vi "Create Evaluation String.vi"(8 "error in (no error)":errorcluster, 10 "Evaluation String":string, 11 "String in":refnum<class "String.lvclass">) -> (0 "error out":errorcluster, 3 "String out":refnum<class "String.lvclass">)   [LabVIEW 2018, in "String.lvclass"]
uses:
  String.lvclass
  Test.lvclass
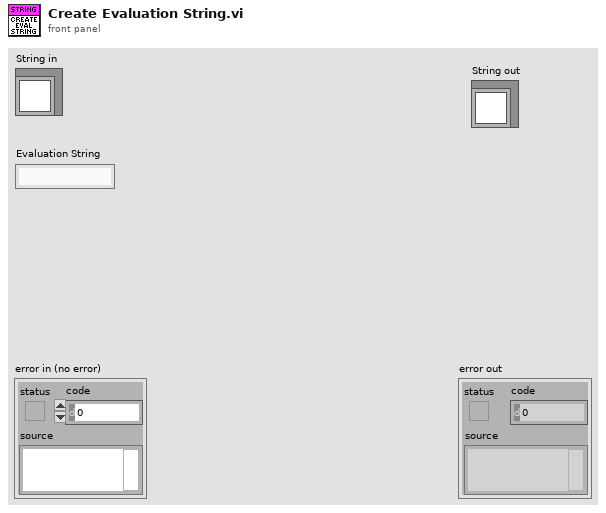
[diagram p1: front panel]
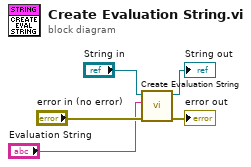
[diagram p0: block diagram]
diagram:
  n1 = call-parent "Create Evaluation String.vi"("error in (no error)"="error in (no error)", "Evaluation String"="Evaluation String", "Test in"="String in") -> ("error out"=→"error out":errorcluster, "Test out"=→"String out":refnum<class "String.lvclass">)  [unwired: 7 in]
